vi "WFS Get Pupil.vi"(8 "error in (no error)":errorcluster {"code" format="%.0x"}, 11 "instrument handle":refnum<visa-resource-name>) -> (0 "error out":errorcluster {"code" format="%.0x"}, 1 "Pupil Center Y mm":dbl, 2 "Pupil Center X mm":dbl, 3 "instrument handle out":refnum<visa-resource-name>, 4 "Pupil Diameter X mm":dbl, 5 "Pupil Diameter Y mm":dbl)   [LabVIEW 2020]
doc: "This VI returns the actual the pupil position and size."
uses:
  WFS_32.dll
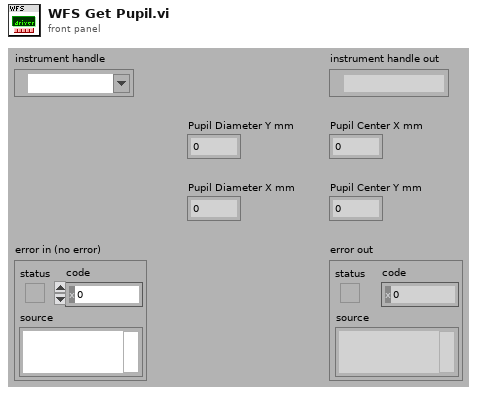
[diagram p1: front panel]
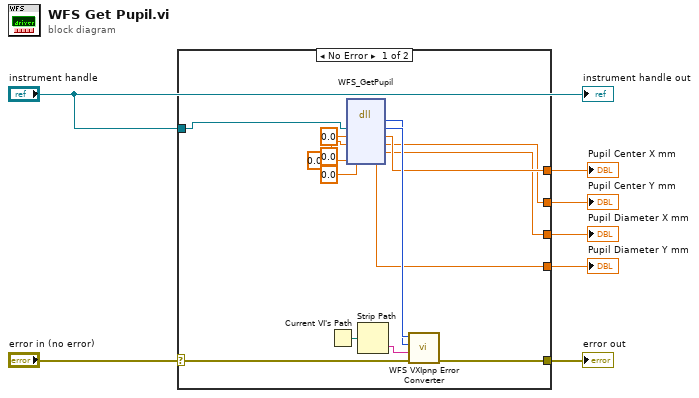
[diagram p0: block diagram]
diagram:
  n1 = case shown="No Error" "error in (no error)" {
    selector: "error in (no error)" -> [w17 w23]
    tunnel: [w16 w23] -> w7
    tunnel: "instrument handle" -> [w21 _]
    tunnel: [w14 _] -> w4
    tunnel: [w12 _] -> w3
    tunnel: [w10 _] -> w2
    tunnel: [w8 _] -> w1
    frame No Error {
      n2 = Current VI's Path() -> (path=w22:path)
      n3 = dll-call lib="WFS_*.*" fn="WFS_GetPupil"("Instrument Handle"=w21, "Pupil Center X mm"=0.0, "Pupil Center Y mm"=0.0, "Pupil Diameter X mm"=0.0, "Pupil Diameter Y mm"=0.0) -> (w19:i32, "Instrument Handle"=w20:u32, "Pupil Center X mm"=w14:dbl, "Pupil Center Y mm"=w12:dbl, "Pupil Diameter X mm"=w10:dbl, "Pupil Diameter Y mm"=w8:dbl)  [unwired: 3 in, 2 out]
      n4 = Strip Path(path=w22) -> (name=w18:string)  [unwired: 1 out]
      n5 = call "WFS VXIpnp Error Converter.vi"("error in (no error)"=w17, "Name Of VI (\"\")"=w18, "CVI Error Code (0)"=w19, "instrument handle"=w20) -> ("error out"=w16:errorcluster)  [unwired: 6 in, 1 out]
    }
    frame Error {
    }
  }
  "error out" <- w7
  "Pupil Center X mm" <- w4
  "Pupil Center Y mm" <- w3
  "Pupil Diameter X mm" <- w2
  "Pupil Diameter Y mm" <- w1
  "instrument handle out" <- "instrument handle"
